vi "get display name.vi"(8 "error in":errorcluster, 11 "protection settings in":refnum<class "protection settings.lvclass">) -> (0 "error out":errorcluster, 2 "class name":string, 3 "protection settings out":refnum<class "protection settings.lvclass">)   [LabVIEW 2013, in "protection settings.lvclass"]
uses:
  protection settings.lvclass
  VI modification.lvclass
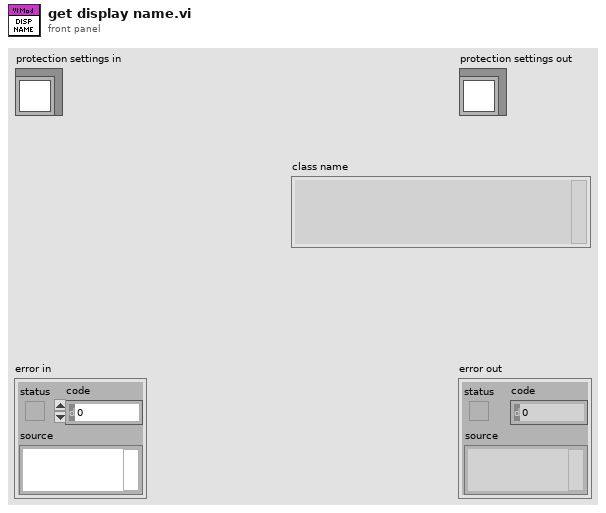
[diagram p1: front panel]
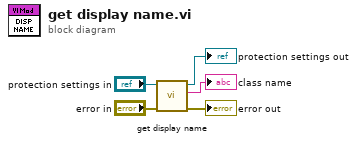
[diagram p0: block diagram]
diagram:
  n1 = call-parent "get display name.vi"("error in"="error in", "VI modification in"="protection settings in") -> ("error out"=→"error out":errorcluster, "class name"=→"class name":string, "VI modification out"=→"protection settings out":refnum<class "protection settings.lvclass">)  [unwired: 7 in]
